vi "Index To Suite.vi"(8 "error in (no error)":errorcluster, 11 "Test Finder In":refnum<class "Test Finder.lvclass">) -> (0 "error out":errorcluster, 2 "Suite":refnum<class "LUnit Test Suite.lvclass">, 3 "Test Finder Out":refnum<class "Test Finder.lvclass">)   [LabVIEW 2020, in "Test Finder.lvclass"]
uses:
  Test Finder.lvclass
  LUnit Test Suite.lvclass
  Test Finder.lvclass/Test Finder.ctl
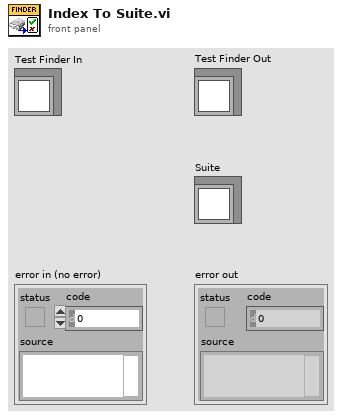
[diagram p1: front panel]
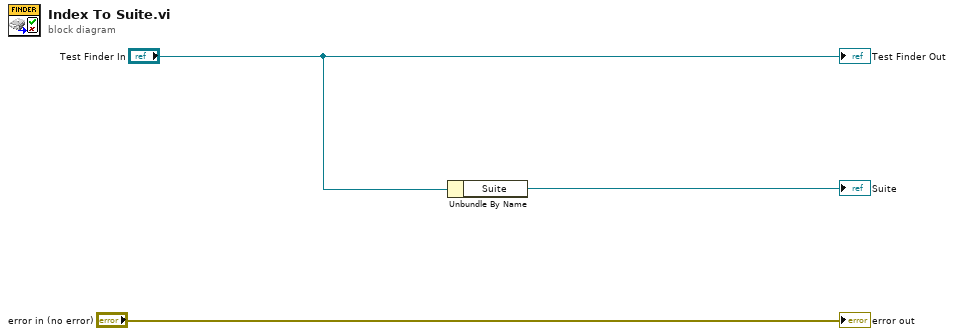
[diagram p0: block diagram]
diagram:
  n1 = Unbundle By Name("Test Finder In") -> ("Suite"=→"Suite":refnum<class "LUnit Test Suite.lvclass">)
  "error out" <- "error in (no error)"
  "Test Finder Out" <- "Test Finder In"
